vi "Make filepath.vi"(8 "error in (no error)":errorcluster, 10 "base path":path, 11 "DAQOrcaFlash in":refnum<class "DAQOrcaFlash.lvclass">) -> (0 "error out":errorcluster, 2 "filepath out":path, 3 "DAQOrcaFlash out":refnum<class "DAQOrcaFlash.lvclass">)   [LabVIEW 2012, in "DAQOrcaFlash.lvclass"]
uses:
  DAQOrcaFlash.lvclass
  DAQOrcaFlash.lvclass/DAQOrcaFlash.ctl
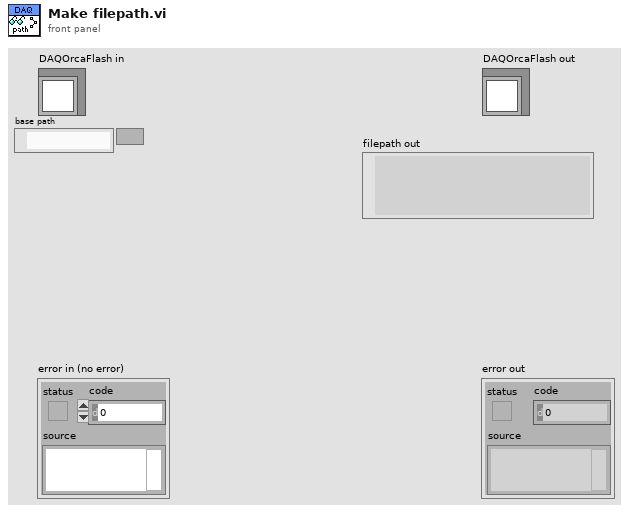
[diagram p1: front panel]
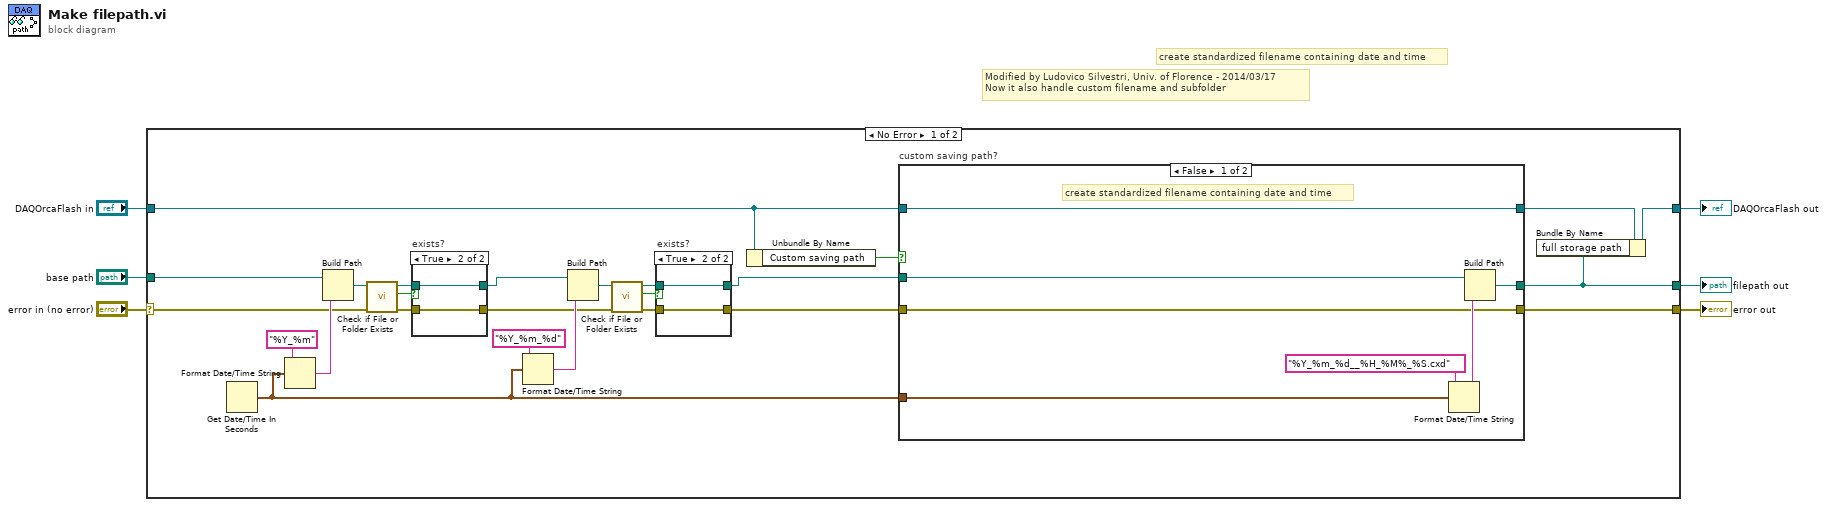
[diagram p0: block diagram]
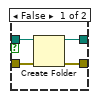
[diagram p2: hidden frame]
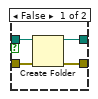
[diagram p3: hidden frame]
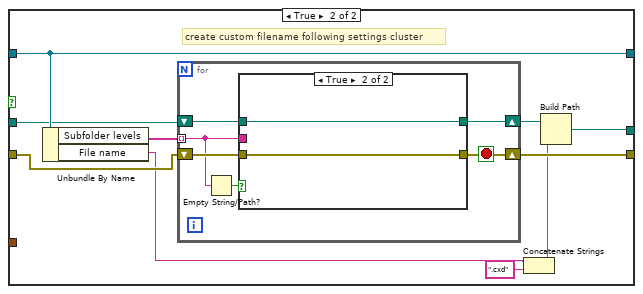
[diagram p4: hidden frame]
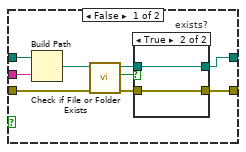
[diagram p5: hidden frame]
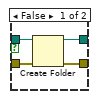
[diagram p6: hidden frame]
diagram:
  # "create standardized filename containing date and time"
  # "Modified by Ludovico Silvestri, Univ. of Florence - 2014/03/17\nNow it also handle custom filename and subfolder"
  n1 = case shown="No Error" "error in (no error)" {
    selector: "error in (no error)" -> [w15 w85]
    tunnel: [w31 w85] -> w5
    tunnel: [w8 w84] -> w4
    tunnel: "DAQOrcaFlash in" -> [w14 w84]
    tunnel: [w7 _] -> w3
    tunnel: "base path" -> [w10 _]
    frame No Error {
      n2 = Get Date/Time In Seconds() -> (seconds since 1Jan1904=w12:timestamp)
      n3 = Format Date/Time String(time format string (%c)="%Y_%m", seconds (now)=w12) -> (date/time string=w29:string)  [unwired: 1 in]
      n4 = Build Path(base path=w10, name or relative path=w29) -> (appended path=w27:path)
      n5 = call <vilib>:"Check if File or Folder Exists.vi"("error in (no error)"=w15, "path"=w27) -> ("error out"=w24:errorcluster, "file or folder exists?"=w26:bool, "dup path"=w25:path)  [unwired: 7 in]
      n6 = case "exists?" shown="True" w26 {
        tunnel: w25 -> [w40 w42]
        tunnel: w24 -> [w41 w43]
        tunnel: [w39 w42] -> w16
        tunnel: [w38 w43] -> w17
        frame False {
          n7 = Create Folder(path (use dialog)=w40, error in=w41) -> (created path=w39:path, error out=w38:errorcluster)  [unwired: 1 in, 1 out]
        }
        frame True {
        }
      }
      n8 = Format Date/Time String(time format string (%c)="%Y_%m_%d", seconds (now)=w12) -> (date/time string=w19:string)  [unwired: 1 in]
      n9 = Build Path(base path=w16, name or relative path=w19) -> (appended path=w23:path)
      n10 = call <vilib>:"Check if File or Folder Exists.vi"("error in (no error)"=w17, "path"=w23) -> ("error out"=w20:errorcluster, "file or folder exists?"=w22:bool, "dup path"=w21:path)  [unwired: 7 in]
      n11 = case "exists?" shown="True" w22 {
        tunnel: w21 -> [w34 w36]
        tunnel: w20 -> [w35 w37]
        tunnel: [w33 w36] -> w11
        tunnel: [w32 w37] -> w13
        frame False {
          n12 = Create Folder(path (use dialog)=w34, error in=w35) -> (created path=w33:path, error out=w32:errorcluster)  [unwired: 1 in, 1 out]
        }
        frame True {
        }
      }
      n13 = Unbundle By Name(w14) -> ("Custom saving path"=w30:bool)
      n14 = case "custom saving path?" shown="False" w30 {
        tunnel: w13 -> [w46 w55]
        tunnel: w14 -> [w49 w60]
        tunnel: [w46 w56] -> w31
        tunnel: [w48 w57] -> w7
        tunnel: [w49 w60] -> w9
        tunnel: w12 -> [w44 _]
        tunnel: w11 -> [w45 w51]
        frame False {
          # "create standardized filename containing date and time"
          n15 = Format Date/Time String(time format string (%c)="%Y_%m_%d__%H_%M%_%S.cxd", seconds (now)=w44) -> (date/time string=w50:string)  [unwired: 1 in]
          n16 = Build Path(base path=w45, name or relative path=w50) -> (appended path=w48:path)
        }
        frame True {
          # "create custom filename following settings cluster"
          n17 = Unbundle By Name(w60) -> ("Subfolder levels"=w59:string[], "File name"=w54:string)
          n18 = for {
            tunnel: w59 -> [w62] mode=indexing
            shift-right: [w64] -> w58
            shift-left: w51 -> [w66]
            shift-right: [w63] -> w56
            shift-left: w55 -> [w65]
            stop <- w63 stop-if-true
            n19 = Empty String/Path?(string/path=w62) -> (empty?=w61:bool)
            n20 = case shown="True" w61 {
              tunnel: w66 -> [w75 w82]
              tunnel: w62 -> [w74 _]
              tunnel: w65 -> [w69 w83]
              tunnel: [w68 w82] -> w64
              tunnel: [w67 w83] -> w63
              frame False {
                n21 = Build Path(base path=w75, name or relative path=w74) -> (appended path=w70:path)
                n22 = call <vilib>:"Check if File or Folder Exists.vi"("error in (no error)"=w69, "path"=w70) -> ("error out"=w73:errorcluster, "file or folder exists?"=w71:bool, "dup path"=w72:path)  [unwired: 7 in]
                n23 = case "exists?" shown="True" w71 {
                  tunnel: w72 -> [w78 w80]
                  tunnel: w73 -> [w79 w81]
                  tunnel: [w77 w80] -> w68
                  tunnel: [w76 w81] -> w67
                  frame False {
                    n24 = Create Folder(path (use dialog)=w78, error in=w79) -> (created path=w77:path, error out=w76:errorcluster)  [unwired: 1 in, 1 out]
                  }
                  frame True {
                  }
                }
              }
              frame True {
              }
            }
          }
          n25 = Concatenate Strings(w54, ".cxd" ("string")) -> (w52:string)
          n26 = Build Path(base path=w58, name or relative path=w52) -> (appended path=w57:path)
        }
      }
      n27 = Bundle By Name(cluster=w9, "full storage path"=w7) -> (w8:refnum<class "DAQOrcaFlash.lvclass">)
    }
    frame Error {
    }
  }
  "error out" <- w5
  "DAQOrcaFlash out" <- w4
  "filepath out" <- w3
